vi "Slope.vi"(1 "X1":dbl, 2 "X2":dbl, 3 "Y1":dbl, 4 "Y2":dbl) -> (0 "Slope":dbl)   [LabVIEW 2020]
panel:
  out "current time":timestamp
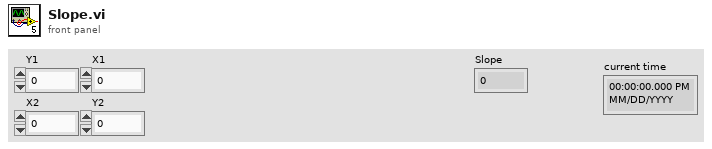
[diagram p1: front panel]
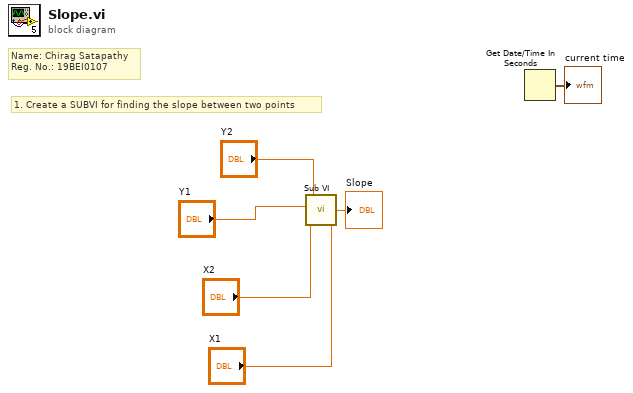
[diagram p0: block diagram]
diagram:
  # "Name: Chirag Satapathy\nReg. No.: 19BEI0107"
  # "1. Create a SUBVI for finding the slope between two points"
  n1 = call "Sub VI.vi"("X1"="X1", "X2"="X2", "Y1"="Y1", "Y2"="Y2") -> ("Slope"=→"Slope":dbl)
  n2 = Get Date/Time In Seconds() -> (seconds since 1Jan1904=→"current time":timestamp)
